vi "Send Command Dispatch.vi"(7 "Message Priority (Normal)":T2=enum."Normal", 8 "error in (no error)":errorcluster, 10 "GUID-cmd-data":T1, 11 "Message Enqueuer":refnum<class "Message Enqueuer.lvclass">) -> (0 "error out":errorcluster, 3 "Message Enqueuer out":refnum<class "Message Enqueuer.lvclass">)   [LabVIEW 2016, in "Controller Actor.lvlib" / "Command Dispatch Msg.lvclass"]
doc: "This VI sends the message to an actor."
uses:
  <userlib>/Common Components/Controller Messages/Command Dispatch Msg/Command Dispatch Msg.lvclass
  <vilib>/ActorFramework/Message Enqueuer/Message Enqueuer.lvclass
  <vilib>/ActorFramework/Message Enqueuer/Message Priority.ctl
  <userlib>/Common Components/Common/GUID-command-data.ctl
  C:/Program Files (x86)/National Instruments/LabVIEW 2016/vi.lib/ActorFramework/Message/Message.lvclass
  <userlib>/Common Components/Controller Messages/Command Dispatch Msg/Command Dispatch Msg.lvclass/Command Dispatch Msg.ctl
  <vilib>/ActorFramework/Message Enqueuer/Message Enqueuer.lvclass/Message Enqueuer.ctl
  <vilib>/ActorFramework/Message Priority Queue/Priority Enqueue.vi
  <userlib>/Common Components/Common/Common.lvlib
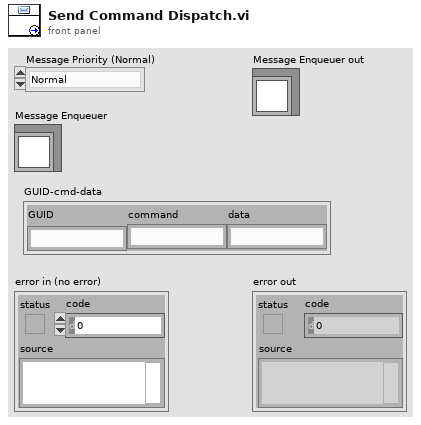
[diagram p1: front panel]
types:
  T1 = typedef "Common.lvlib/GUID-command-data.ctl" = cluster{"GUID":string, "command":string, "data":string}
  T2 = typedef "Actor Framework.lvlib/Message Enqueuer.lvclass/Message Priority.ctl" = enum16{"Low", "Normal", "High"}
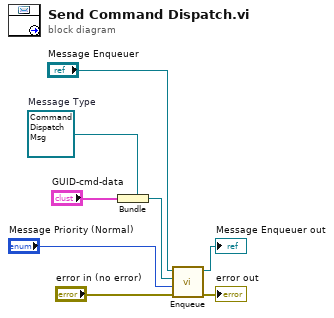
[diagram p0: block diagram]
diagram:
  w5 = refnum<class "Command Dispatch Msg.lvclass"> refnum  # Message Type
  n1 = Bundle(cluster=w5, "GUID-cmd-data") -> (w4:refnum<class "Command Dispatch Msg.lvclass">)
  n2 = call <vilib>:"Enqueue.vi"("error in (no error)"="error in (no error)", "Message Priority (Normal)"="Message Priority (Normal)", "Message"=w4, "Message Enqueuer in"="Message Enqueuer") -> ("error out"=→"error out":errorcluster, "Message Enqueuer out"=→"Message Enqueuer out":refnum<class "Message Enqueuer.lvclass">)  [unwired: 6 in]
